vi "Train Wheel PtByPt.vi"() -> ()   [LabVIEW 2023]
doc: "Simulated real-world application of Point By Point. Detects train wheel defects based on simulated real-time data acquisition and analysis. Each train has 6 wheels and is each wheel is represented by a spike in the chart of the Simulated data. The height of the spike determines whether the wheel is good. After each train passes the bar graph at the bottom shows how good each of the wheels are."
uses:
  <vilib>/Analysis/3filter.llb/Filter Passband Type.ctl
  <vilib>/ptbypt/NI_PtbyPt.lvlib
  <vilib>/Analysis/NI_AALBase.lvlib
panel:
  in  "Tab Control":enum32{"Introduction", "Signal"}(tab)
  out "Train detected":bool
  out "Threshold Data":dbl(graph)
  out "Simulated Data (8 trains)":cluster{"Filtered x":dbl, dbl, "threshold":dbl}(graph)
  out "Bad/Good Wheels":dbl[](graph)
  out "no. of train":u32
  out "Wheel detected":bool
  out "no. of wheel":u32
  in  "Filter  order":i32=4
  in  "Low Frequency":dbl=0.01 format="%#.6g"
  in  "Window length":i32=100
  in  "Threshold":dbl(slide)=15.0 scale=-10.0..40.0
  in  "High Frequency":dbl=0.25 format="%#.6g"
  in  "Simulation Speed":u32(slide)=5 scale=1.0..10.0
  in  "Stop":bool
  # "Magnetic Sensor"
  # "Overview: In this example, the maintenance staff of a train yard must detect defective wheels on a train. The current method of detection consists of a railroad worker striking a wheel with a hammer and listening for a different resonance that identifies a flaw. Automated surveillance must replace manual testing, because manual surveillance is too slow, too prone to error, and too crude to detect subtle defects. An automated solution also adds the power of dynamic testing, because the train wheels can be in service during the test, instead of standing still. The point-by-point detection application must analyze the low- and high-frequency components separately. The Array Max & Min PtByPt VI extracts waveform data that reveals the level of energy in the waveform for each wheel, the end of each train, and the end of each wheel.\nRequirements: LabVIEW Full Development System\nInstructions:\n1. Run the VI.\n2. Verify that when the wheel passes over the magnetic sensor, a spike is captured.\n3. Change values on the Signal tab to see the effect different configurations have on the analysis.\n4. Click Stop to stop the VI."
  # "Filter Parameters"
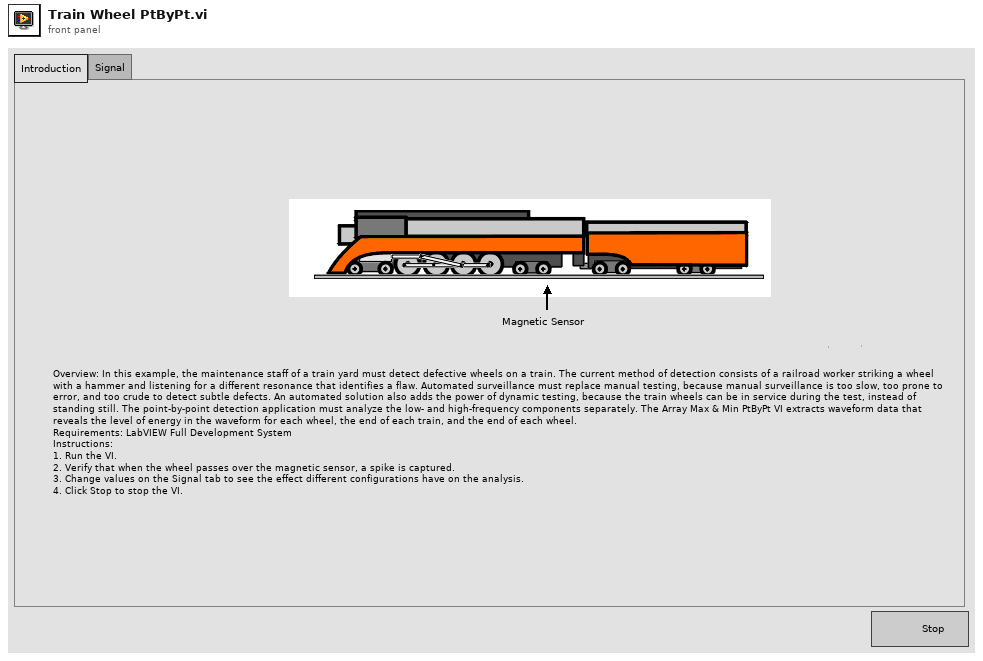
[diagram p1: front panel]
types:
  T1 = cluster{dbl, "Filtered x":dbl, "Filtered x 2":dbl}[]
  T2 = typedef "NI_AALBase.lvlib/Filter Passband Type.ctl" = enum32{"Lowpass", "Highpass", "Bandpass", "Bandstop"}
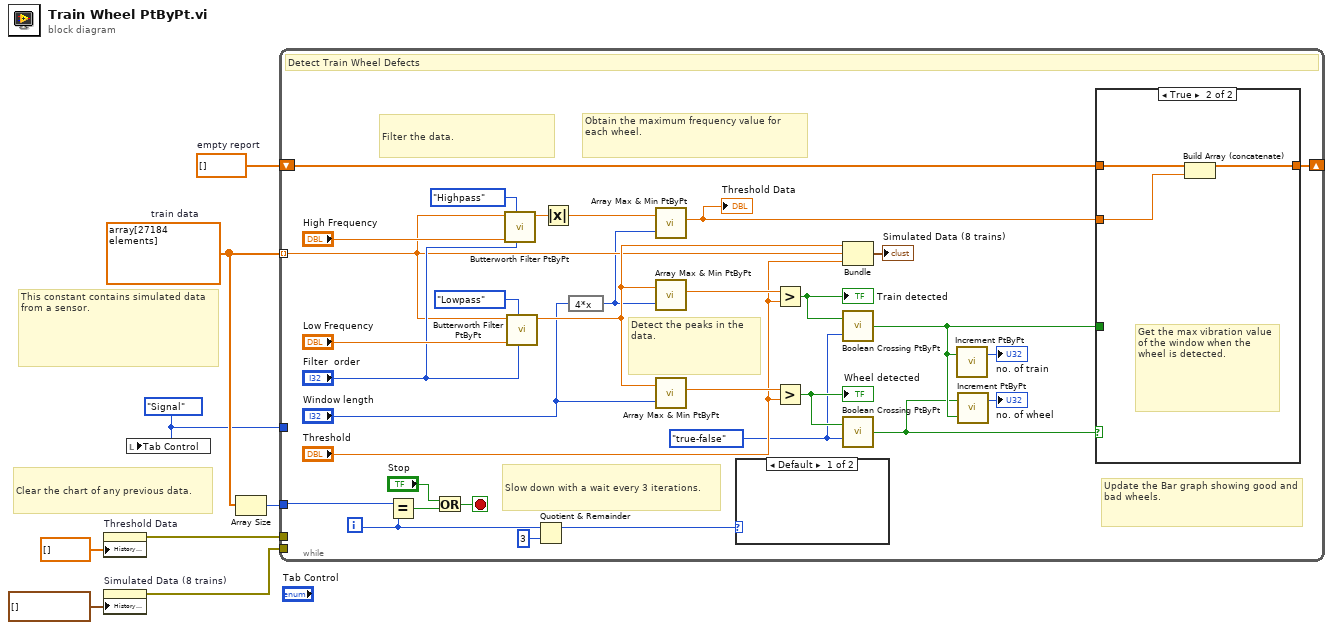
[diagram p0: block diagram]
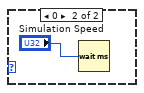
[diagram p2: hidden frame]
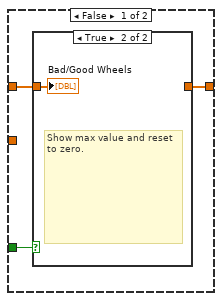
[diagram p3: hidden frame]
diagram:
  w1 = enum32{"Introduction", "Signal"}."Signal" ("Tab Control")
  w6 = dbl[] array[27184 elements]  # train data
  w8 = dbl[] []  # empty report
  # "Clear the chart of any previous data."
  # "This constant contains simulated data from a sensor."
  n1 = property on="Threshold Data" class="WFChart (strict)"("History Data"=dbl[] []) -> (error out=w5:errorcluster)  [unwired: 2 in, 1 out]
  n2 = property on="Simulated Data (8 trains)" class="WFChart (strict)"("History Data"=T1 []) -> (error out=w2:errorcluster)  [unwired: 2 in, 1 out]
  n3 = local write "Tab Control"(w1) -> ()
  n4 = Array Size(array=w6) -> (size(s)=w7:i32)
  n5 = while {
    shift-left: w8 -> [w35]
    shift-right: [w36] -> _
    tunnel: w6 -> [w21] mode=indexing
    tunnel: w5 -> [_]
    tunnel: w7 -> [w30]
    tunnel: w2 -> [_]
    tunnel: w1 -> [_]
    i -> [w29]
    stop <- w31 stop-if-true
    w9 = enum16{"either", "false-true", "true-false"}."true-false" ("direction")
    # "Update the Bar graph showing good and bad wheels."
    # "Detect the peaks in the data."
    # "Obtain the maximum frequency value for each wheel."
    # "Filter the data."
    # "Slow down with a wait every 3 iterations."
    # "Detect Train Wheel Defects"
    n6 = Equal?(x=w30, y=w29) -> (x = y?=w25:bool)
    n7 = Or(x="Stop", y=w25) -> (x .or. y?=w31:bool)
    n8 = call <vilib>:"Butterworth Filter PtByPt.vi"("order"="Filter  order", "filter type"=Filter_Passband_Type."Highpass", "low cutoff freq: fl"="High Frequency", "x"=w21) -> ("Filtered x"=w13:dbl)  [unwired: 5 in, 1 out]
    n9 = call <vilib>:"Butterworth Filter PtByPt.vi"("order"="Filter  order", "filter type"=Filter_Passband_Type."Lowpass", "low cutoff freq: fl"="Low Frequency", "x"=w21) -> ("Filtered x"=w22:dbl)  [unwired: 5 in, 1 out]
    n10 = Quotient & Remainder(x=w29, y=3) -> (x-y*floor(x/y)=w27:i32)  [unwired: 1 out]
    n11 = Absolute Value(x=w13) -> (abs(x)=w23:dbl)
    n12 = expression code="4*x"("Window length") -> (w14:i32)
    n13 = call <vilib>:"Array Max & Min PtByPt.vi"("input data point"=w23, "sample length"=w14) -> ("max value"=w12:dbl)  [unwired: 1 in, 4 out]
    "Threshold Data" <- w12
    n14 = call <vilib>:"Array Max & Min PtByPt.vi"("input data point"=w22, "sample length"=w14) -> ("max value"=w34:dbl)  [unwired: 1 in, 4 out]
    n15 = call <vilib>:"Array Max & Min PtByPt.vi"("input data point"=w22, "sample length"="Window length") -> ("max value"=w37:dbl)  [unwired: 1 in, 4 out]
    n16 = case shown="Default" w27 {
      frame Default {
      }
      frame 0 {
        n17 = Wait (ms)(milliseconds to wait="Simulation Speed") -> ()  [unwired: 1 out]
      }
    }
    n18 = Greater?(x=w34, y="Threshold") -> (0:w17:bool)
    "Train detected" <- w17
    n19 = Greater?(x=w37, y="Threshold") -> (0:w16:bool)
    "Wheel detected" <- w16
    n20 = Bundle("Filtered x"=w22, w21, "Threshold"="Threshold") -> (→"Simulated Data (8 trains)":cluster{"Filtered x":dbl, dbl, "Threshold":dbl})  [unwired: 1 in]
    n21 = call <vilib>:"Boolean Crossing PtByPt.vi"("direction"=w9, "input"=w17) -> ("crossing"=w19:bool)  [unwired: 1 in]
    n22 = call <vilib>:"Boolean Crossing PtByPt.vi"("direction"=w9, "input"=w16) -> ("crossing"=w18:bool)  [unwired: 1 in]
    n23 = call <vilib>:"Increment PtByPt.vi"("activate"=w19) -> ("counter"=→"no. of train":u32)  [unwired: 1 in, 1 out]
    n24 = call <vilib>:"Increment PtByPt.vi"("initialize"=w19, "activate"=w18) -> ("counter"=→"no. of wheel":u32)  [unwired: 1 out]
    n25 = case shown="True" w18 {
      tunnel: w12 -> [_ w47]
      tunnel: w19 -> [w44 _]
      tunnel: [w43 w48] -> w36
      tunnel: w35 -> [w42 w49]
      frame False {
        n26 = case shown="True" w44 {
          tunnel: [w45 _] -> w43
          tunnel: w42 -> [w45 w46]
          frame False {
          }
          frame True {
            # "Show max value and reset to zero."
            "Bad/Good Wheels" <- w46
          }
        }
      }
      frame True {
        # "Get the max vibration value of the window when the wheel is detected."
        n27 = Build Array (concatenate)(w49, w47) -> (w48:dbl[])
      }
    }
  }
